vi "Global - Handle.vi"() -> ()   [LabVIEW 2019]
panel:
  in  "Handle":T1(array[cluster])
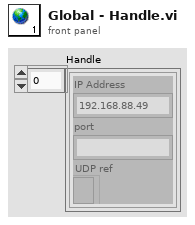
[diagram p1: front panel]
types:
  T1 = cluster{"IP Address":string, "port":string, "UDP ref":refnum<k16>}[]
diagram:
